vi "TCP_NoDelay_Windows.vi"(4 "error in (no error)":errorcluster, 6 "TCP_NODELAY (true)":bool=TRUE, 7 "connID":refnum<k5>) -> (0 "error out":errorcluster, 3 "connID 2":refnum<k5>)   [LabVIEW 2018]
doc: "This VI takes a LabVIEW TCP Connection ID and either sets or clears the TCP_NODELAY flag on the underlying socket. Upon creation of a socket this flag is by default clear, meaning that the Nagle algorithm is in effect. By setting the TCP_NODELAY flag, the Nagle algorithm is disabled for the given connection. \n\nYou should disable the Nagle algorithm with care - it is one of the basic algorithms of TCP that helps reduce internet traffic by coalescing several small packets into a single large one. However, sometimes disabling it is useful in reducing latency in protocols that have a query/response nature.\n\nFor more information on the Nagle algorithm, google \"nagle\".\nFor platform specific notes, see the diagram."
uses:
  wsock32.dll
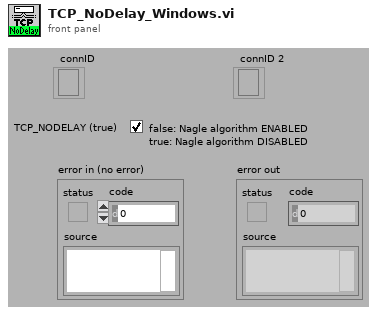
[diagram p1: front panel]
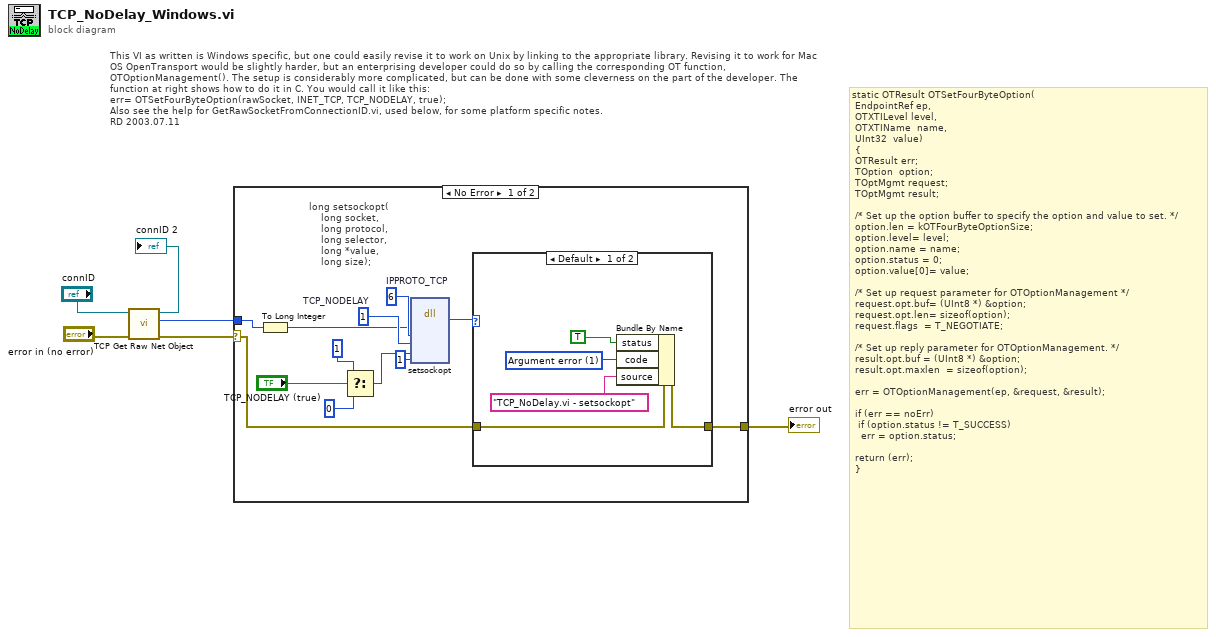
[diagram p0: block diagram]
diagram:
  # "static OTResult OTSetFourByteOption(\n\tEndpointRef ep,\n\tOTXTILevel level,\n\tOTXTIName  name,\n\tUInt32\t value)\n\t{\n\tOTResult err;\n\tTOption  option;\n\tTOptMgmt request;\n\tTOptMgmt result;\n\n\t/* Set up the option buffer to specify the option and value to set. */\n\toption.len\t= kOTFourByteOptionSize;\n\toption.level= level;\n\toption.name = name;\n\toption.status = 0;\n\toption.value[0]= value;\n\n\t/* Set up request parameter for OTOptionManagement */\n\trequest.opt.buf= (UInt8 *) &option;\n\trequest.opt.len= sizeof(option);\n\trequest.flags  = T_NEGOTIATE;\n\n\t/* Set up reply parameter for OTOptionManagement. */\n\tresult.opt.buf\t= (UInt8 *) &option;\n\tresult.opt.maxlen  = sizeof(option);\n\n\terr = OTOptionManagement(ep, &request, &result);\n\n\tif (err == noErr)\n\t\tif (option.status != T_SUCCESS)\n\t\t\terr = option.status;\n\n\treturn (err);\n\t}"
  # "This VI as written is Windows specific, but one could easily revise it to work on Unix by linking to the appropriate library. Revising it to work for Mac OS OpenTransport would be slightly harder, but an enterprising developer could do so by calling the corresponding OT function, OTOptionManagement(). The setup is considerably more complicated, but can be done with some cleverness on the part of the developer. The function at right shows how to do it in C. You would call it like this:\nerr= OTSetFourByteOption(rawSocket, INET_TCP, TCP_NODELAY, true);\nAlso see the help for GetRawSocketFromConnectionID.vi, used below, for some platform specific notes.\nRD 2003.07.11"
  n1 = call <vilib>:"TCP Get Raw Net Object.vi"("error in (no error)"="error in (no error)", "connection ID"="connID") -> ("error out"=w5:errorcluster, "raw net object"=w3:u64, "connection ID out"=→"connID 2":refnum<k5>)  [unwired: 7 in]
  n2 = case shown="No Error" w5 {
    selector: w5 -> [w8 w25]
    tunnel: [w10 w25] -> w6
    tunnel: w3 -> [w9 _]
    frame No Error {
      w17 = 1  # TCP_NODELAY
      w18 = 6  # IPPROTO_TCP
      # "long setsockopt(\n    long socket,\n    long protocol,\n    long selector,\n    long *value,\n    long size);"
      n3 = To Long Integer(number=w9) -> (32bit integer=w7:i32)
      n4 = Select(t=i8 1, s="TCP_NODELAY (true)", f=i8 0) -> (s? t:f=w14:i8)
      n5 = dll-call lib="wsock32.dll" fn="setsockopt" ("Call Library Function")("socket"=w7, "protocol"=w18, "selector"=w17, "value"=w14, "size"=1) -> (w11:i32)  [unwired: 8 in, 2 out]
      n6 = case shown="Default" w11 {
        tunnel: [w23 w24] -> w10
        tunnel: w8 -> [w19 w24]
        frame Default {
          w22 = 1 items=["No error", "Argument error", "Memory is full", "Out of zone", "End of file", "File already open", "Generic file I/O error", "File not found", "File permission error", "Disk is full", "Duplicate path", "Too many files open", "System feature not enabled", "Resource file not found", "Cannot add resource", "Resource not found", "Image not found", "Image memory error", "Pen does not exist", "Config type invalid", "Config token not found", "Config parse error", "Config memory error", "Bad external code format", "Bad external code offset", "External code not present", "Null window", "Destroy window error", "Null menu", "Print aborted", "Bad print record", "Print driver error", "Windows error during printing", "Memory error during printing", "Print dialog error", "Generic print error", "Invalid device refnum", "Device not found", "Device parameter error", "Device unit error", "Cannot open device", "Device call aborted", "Generic error", "Cancelled by user", "Object ID too low", "Object ID too high", "Object not in heap", "Unknown heap", "Unknown object (invalid DefProc)", "Unknown object (DefProc not in table)", "Message out of range", "Invalid (null) method", "Unknown message", "Manager call not supported", "Bad address", "Network operation in progress", "Network operation timed out", "Connection is busy", "Network attribute not supported", "Network error", "Address in use", "System out of memory", "Connection aborted", "Connection refused", "Not connected", "Already connected", "Connection closed", "Initialization error (interapplication manager)", "Bad occurrence", "Wait on unbound occurrence handler", "Occurrence queue overflow", "Datalog type conflict", "Unused", "Unrecognized type (interapplication manager)", "Memory corrupt", "Failed to make temporary DLL", "Old CIN version", "Drag socket not found", "Failed to load drop-object", "Failed to register OLE object", "Failed to release OLE object", "Format specifier type mismatch", "Unknown format specifier", "Too few format specifiers", "Too many format specifiers", "Scan failed", "Newer CIN version", "Error converting to variant", "Runtime menu error", "Password tampered", "Variant attribute not found", "Incompatible variant data type", "Event data is not available", "Event Store is not present", "Occurrence is not found", "Event Queue is not created", "Event info is not available", "Refnum passed is NULL", "Error retrieving Class GUID", "Error retrieving CoClass GUID", "Error retrieving TypeLib GUID.", "Bad built application magic bytes.", "Specific driver is different from the specific driver associated with the Logical Name.", "There is no session opened to the class driver.", "Max Error", "MAX - Error with config objects", "MAX - Error loading configuration", "MAX - Group not supported"]
          n7 = Bundle By Name(cluster=w19, "status"=TRUE, "code"=w22, "source"="TCP_NoDelay.vi - setsockopt") -> (w23:errorcluster)
        }
        frame 0 {
        }
      }
    }
    frame Error {
    }
  }
  "error out" <- w6
